vi "Process.vi"(8 "error in":errorcluster, 11 "Logger.Error":refnum<class "Logger.Error.lvclass">) -> (0 "error out":errorcluster, 3 "Logger.Error out":refnum<class "Logger.Error.lvclass">)   [LabVIEW 2019, in "Logger.Error.lvlib" / "Logger.Error.lvclass"]
doc: "---------------------------------------------------------------\nJKI State Machine Objects™\nhttp://jki.net/state-machine-objects/\nCopyright (C) 2005-2015, JKI <info@jki.net>\nALL RIGHTS RESERVED"
uses:
  Logger.Error.lvclass
  C:/Program Files/National Instruments/LabVIEW 2019/vi.lib/JKI/JKI SMO/SMO/SMO.lvclass
  Logger.Error.lvclass/Logger.Error.ctl
  <vilib>/JKI/JKI SMO/SMO/SMO.lvclass/SMO.ctl
  e2013399-adaa-4ae5-b634-22c116f18404.vi
  <vilib>/JKI/JKI SMO/SMO/Private/ReftoDVR--SMO.vi
  <vilib>/Utility/file.llb/Write Delimited Spreadsheet (string).vi
  <userlib>/LevyLab/Logger/Logger/Logger.lvclass
  <userlib>/LevyLab/Debug/Debug.lvlib
  <vilib>/JKI/JKI SMO/SMO/SMO.lvclass
panel:
  out "Status":string
  out "State History":string
  # "error Logger"
  # "For instructions on how to use the JKI State Machine Objects, examples and video tutorials, visit:\nhttp://jki.net/state-machine-objects/\n\nJKI State Machine Objects™\nhttp://jki.net/state-machine-objects/\nCopyright (C) 2005-2015, JKI <info@jki.net>\nALL RIGHTS RESERVED"
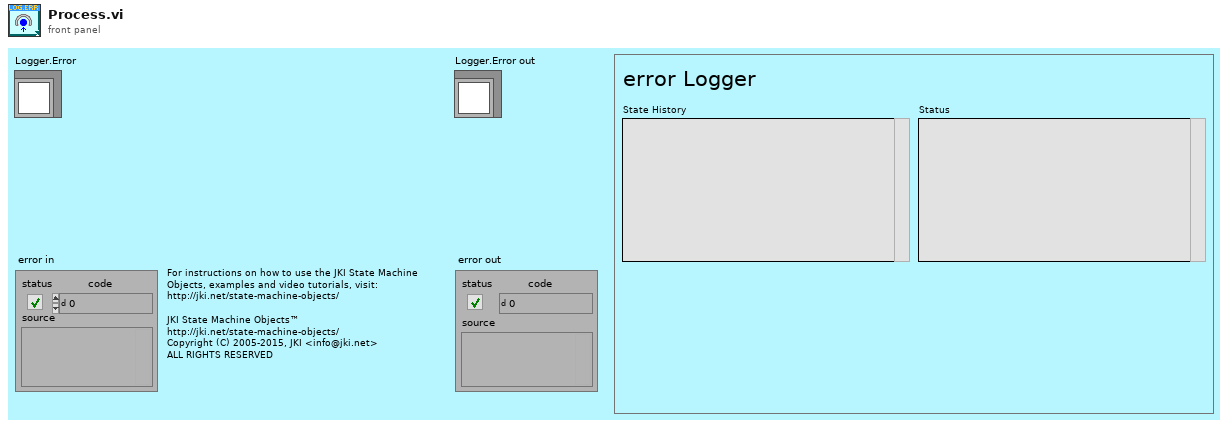
[diagram p1: front panel]
types:
  T1 = enum32{"invalid app kind", "Development System", "Run Time System", "Student Edition", "Embedded LabVIEW", "Evaluation", "Custom"}
  T2 = enum32{"Invalid", "Standard", "Closed", "Hidden", "Minimized", "Maximized"}
  T3 = cluster{"Core":cluster{"Current VI Reference":refnum<vi>, "Close Panel on Exit?":bool, "Last Error":cluster{"error":errorcluster, "previous state":string, "remaining states":string}, "Shutdown?":bool}, "SelfRef":refnum<class "Logger.Error.lvclass">, "path":path, "SMOs":refnum<class "SMO.lvclass">[], "error to log":errorcluster}
  T4 = cluster{"Current VI Reference":refnum<vi>, "Close Panel on Exit?":bool, "Last Error":cluster{"error":errorcluster, "previous state":string, "remaining states":string}, "Shutdown?":bool}
  T5 = typedef "Debug.lvlib/Attribute.Debug.lvclass/DebugBehavior.ctl" = enum16{"Normal", "Debug"}
  T6 = typedef "SMO.lvclass/Protected Events.ctl" = cluster{"StopProcesses":refnum<user-event>, "AbortProcesses":refnum<user-event>, "Config Changed":refnum<user-event>, "Dependency":refnum<user-event>}
  T7 = typedef "SMO.lvclass/Public Events.ctl" = cluster{"Error":refnum<user-event>, "State":refnum<user-event>, "Reserve State":refnum<user-event>}
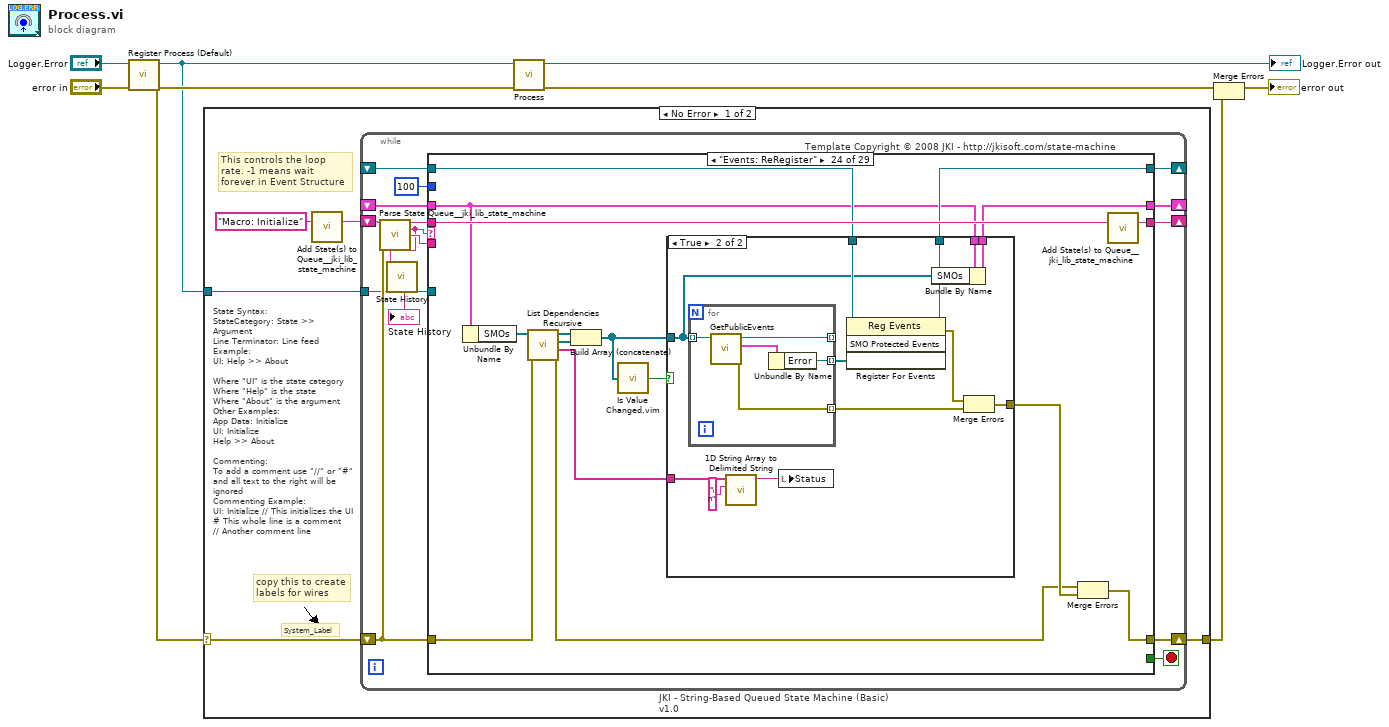
[diagram p0: block diagram]
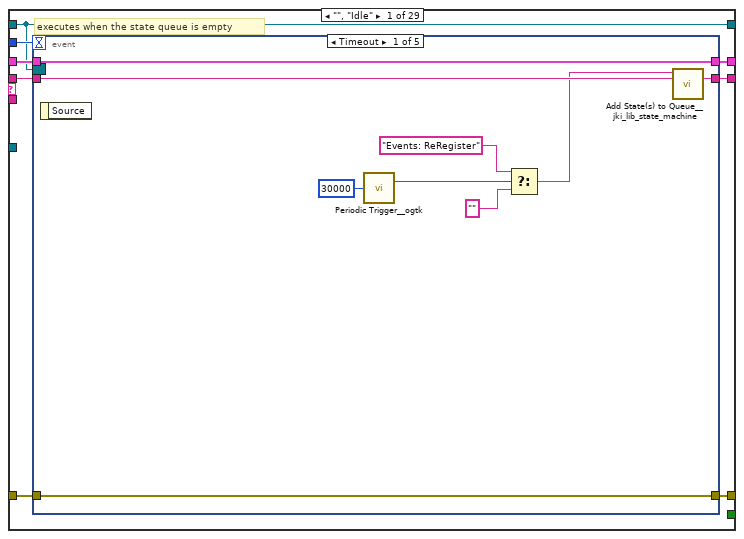
[diagram p2: hidden frame]
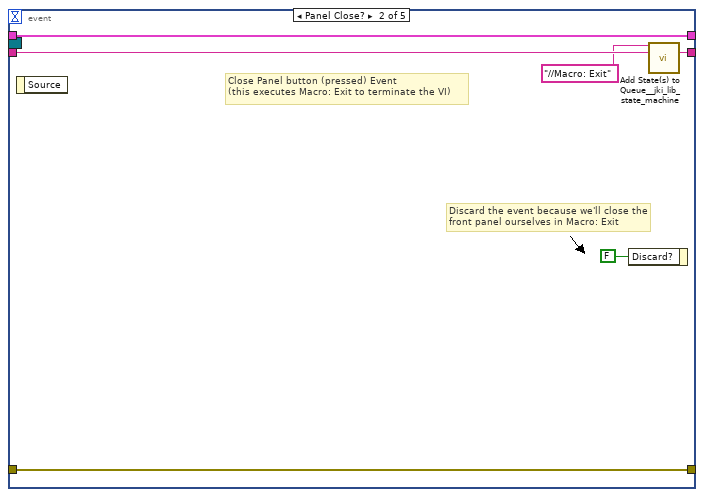
[diagram p3: hidden frame]
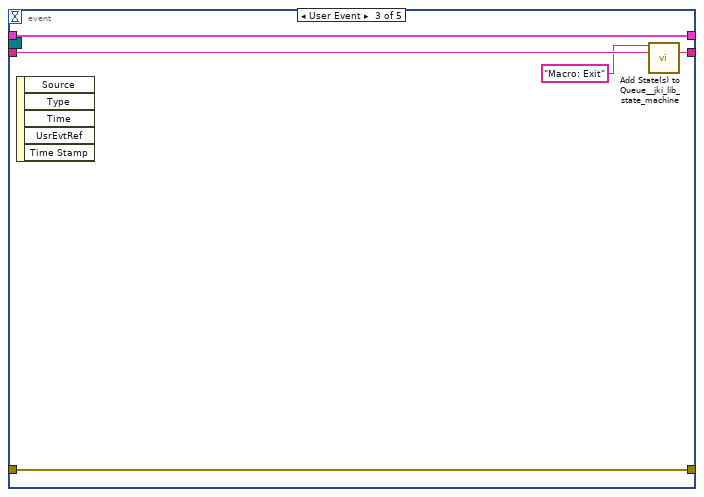
[diagram p4: hidden frame]
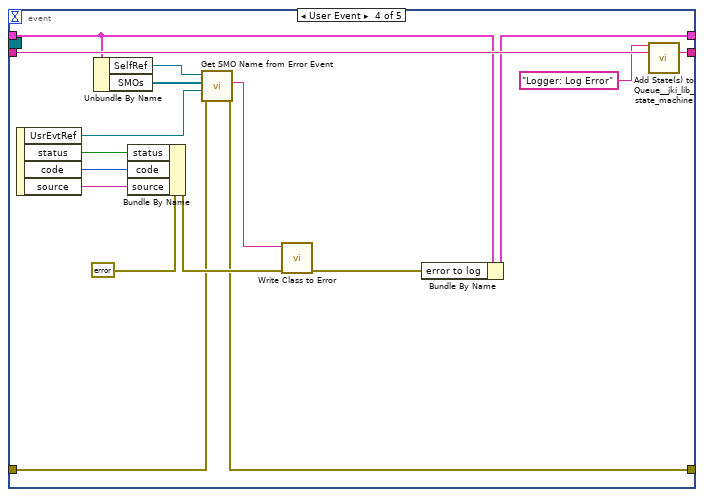
[diagram p5: hidden frame]
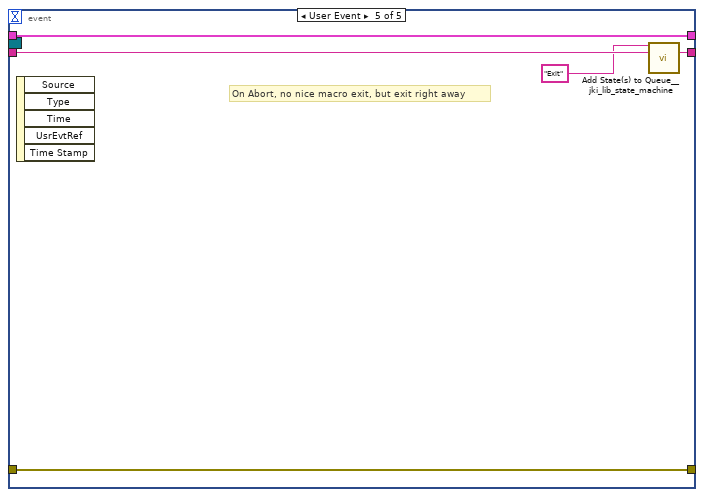
[diagram p6: hidden frame]
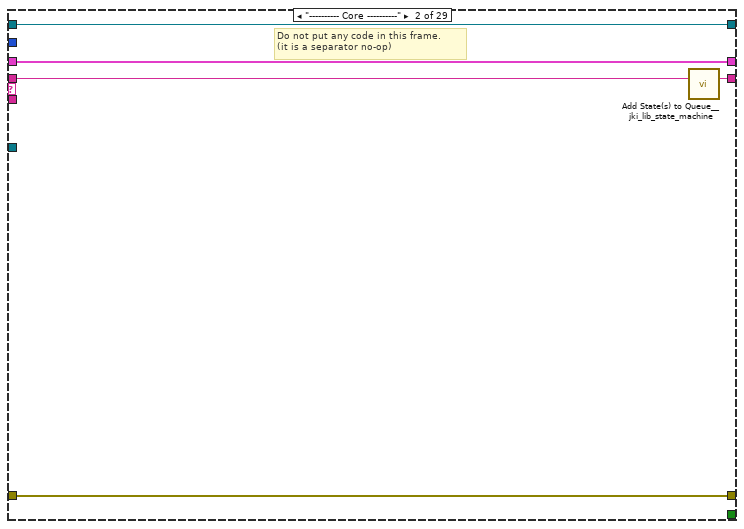
[diagram p7: hidden frame]
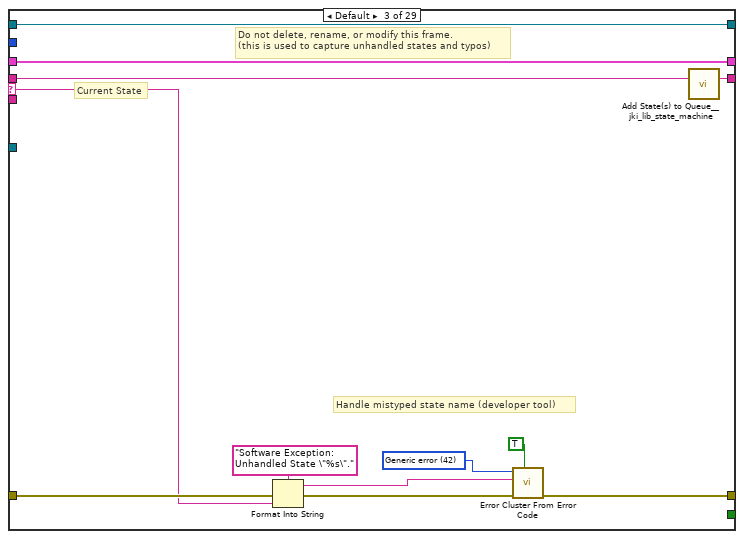
[diagram p8: hidden frame]
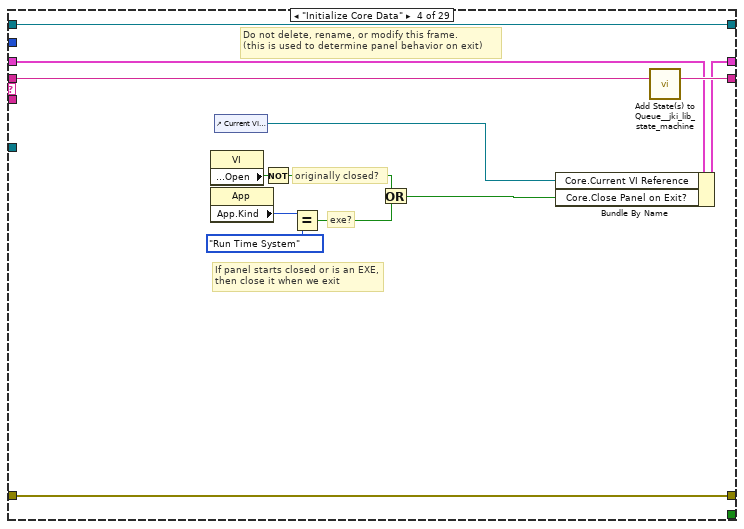
[diagram p9: hidden frame]
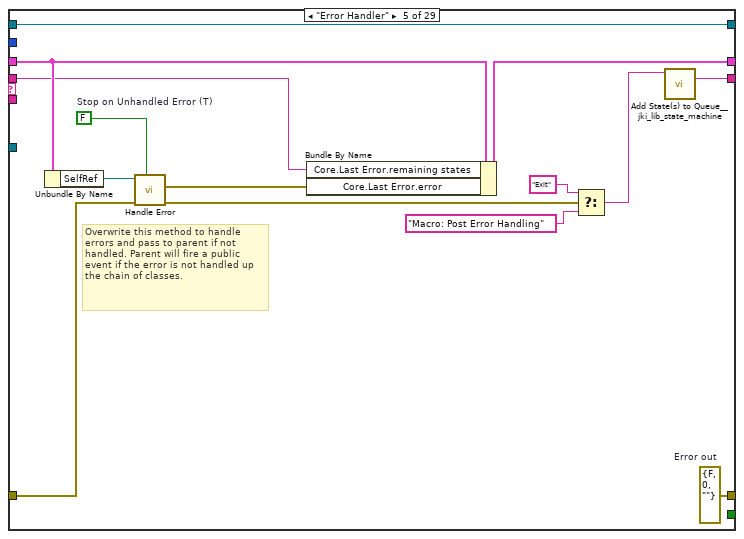
[diagram p10: hidden frame]
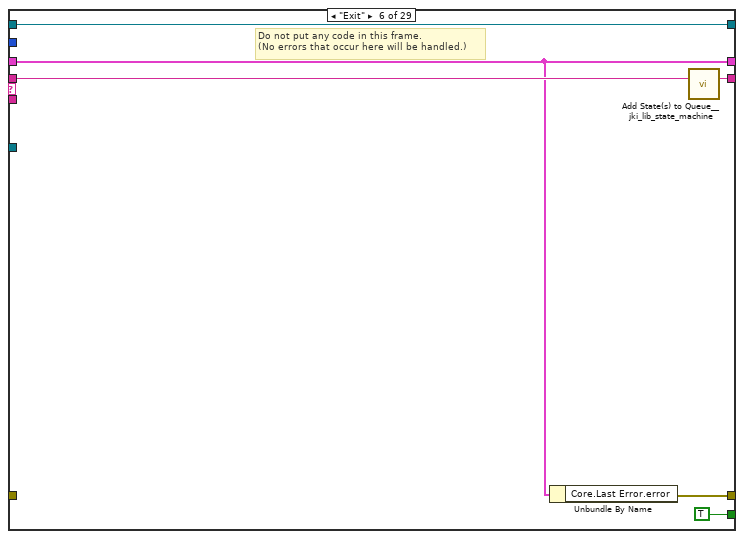
[diagram p11: hidden frame]
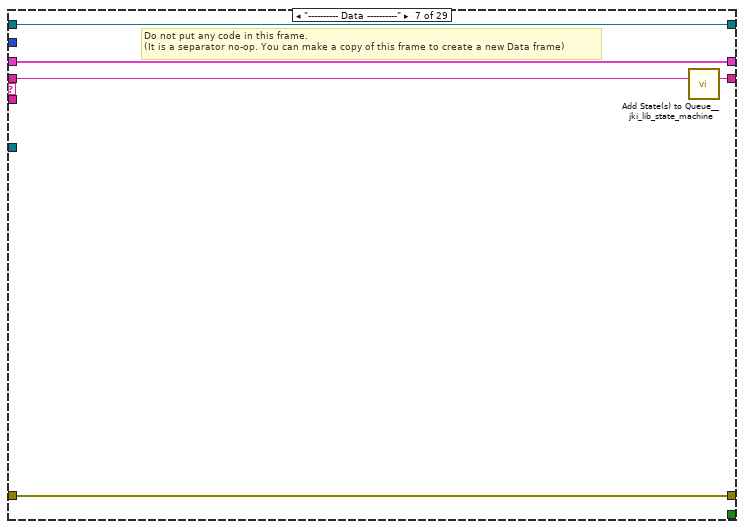
[diagram p12: hidden frame]
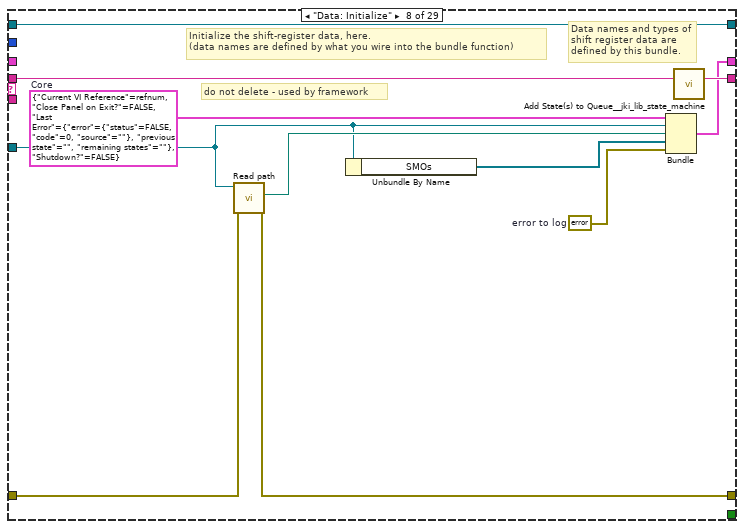
[diagram p13: hidden frame]
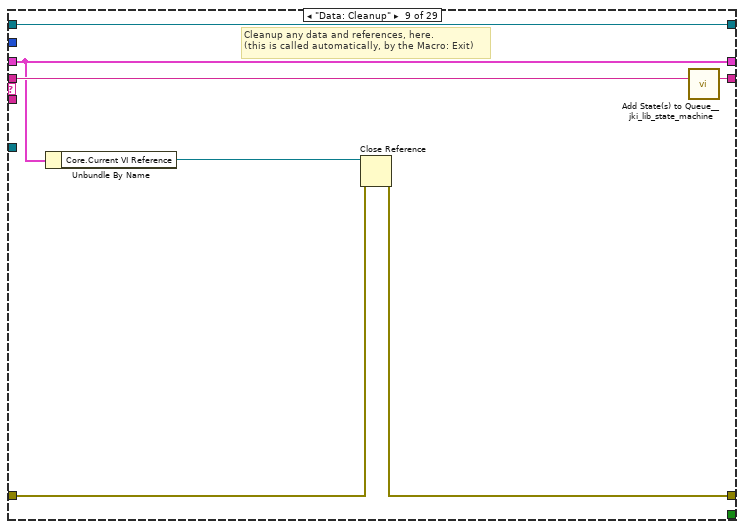
[diagram p14: hidden frame]
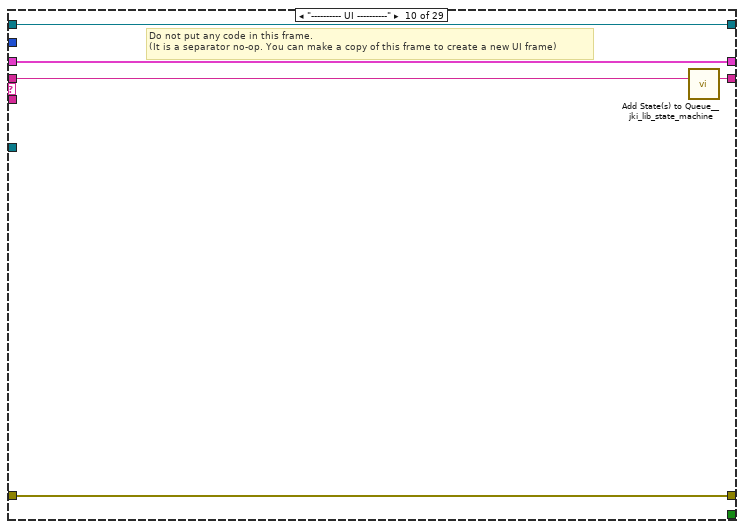
[diagram p15: hidden frame]
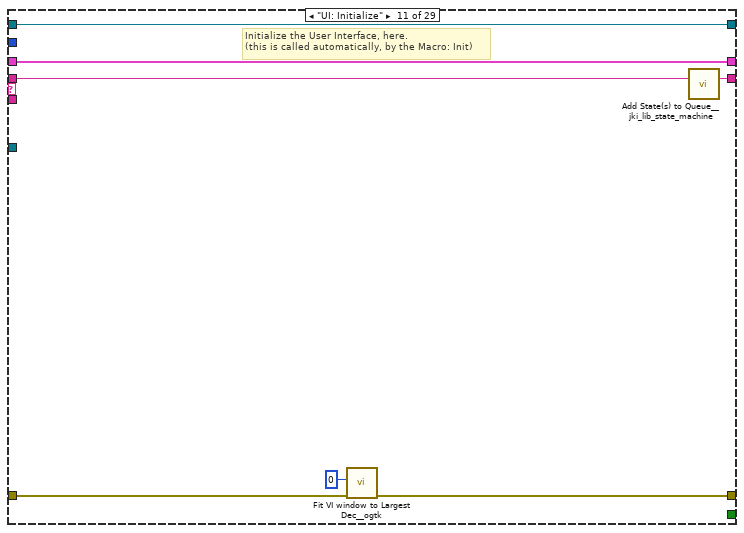
[diagram p16: hidden frame]
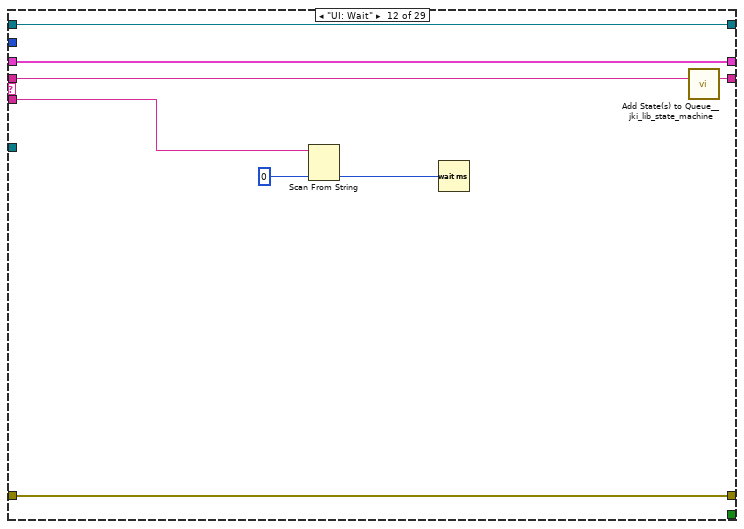
[diagram p17: hidden frame]
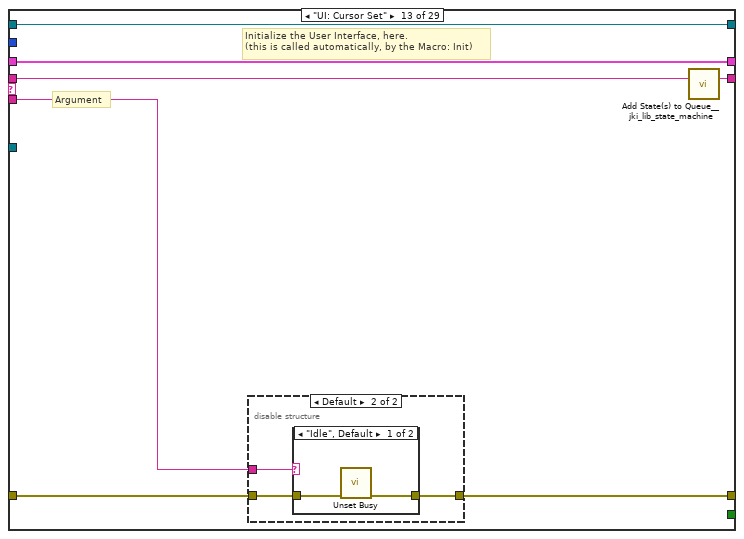
[diagram p18: hidden frame]
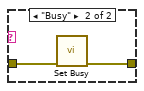
[diagram p20: hidden frame]
diagram:
  n1 = call <vilib>:"Register Process (Default).vi"("error in (no error)"="error in", "SMO"="Logger.Error") -> ("error out"=w5:errorcluster, "SelfRef"=w4:refnum<class "Logger.Error.lvclass">)  [unwired: 8 in]
  n2 = case shown="No Error" w5 {
    selector: w5 -> [w10 w420]
    tunnel: w4 -> [w11 _]
    tunnel: [w9 w420] -> w1
    frame No Error {
      # "State Syntax:\nStateCategory: State >> Argument\nLine Terminator: Line feed\nExample:\nUI: Help >> About\n\nWhere \"UI\" is the state category\nWhere \"Help\" is the state\nWhere \"About\" is the argument\nOther Examples:\nApp Data: Initialize\nUI: Initialize\nHelp >> About\n\nCommenting:\nTo add a comment use \"//\" or \"#\" and all text to the right will be ignored\nCommenting Example:\nUI: Initialize // This initializes the UI\n# This whole line is a comment\n// Another comment line"
      # "copy this to create labels for wires"
      # "This controls the loop rate. -1 means wait forever in Event Structure"
      # "System_Label"
      n3 = call <vilib>:"Add State(s) to Queue__jki_lib_state_machine.vi"("State(s) in (\"\")"="Macro: Initialize") -> ("States Out"=w13:string)  [unwired: 14 in]
      n4 = while "JKI - String-Based Queued State Machine (Basic) v1.0" {
        shift-right: [w22] -> _
        shift-left: _ -> [w14]
        shift-right: [w25] -> w9
        shift-left: w10 -> [w20]
        shift-right: [w24] -> _
        shift-left: w13 -> [w26]
        tunnel: w11 -> [w19]
        shift-right: [w18] -> _
        shift-left: _ -> [w17]
        stop <- w23 stop-if-true
        # "Template Copyright © 2008 JKI - http://jkisoft.com/state-machine"
        n5 = call <vilib>:"Parse State Queue__jki_lib_state_machine.vi"("State Queue"=w26, "Error In (no error)"=w20) -> ("Remaining States"=w28:string, "Current State"=w15:string, "Arguments"=w27:string)  [unwired: 11 in]
        n6 = call <userlib>:"State History.vi"("Current State"=w15) -> ("History"=→"State History":string)  [unwired: 10 in]
        n7 = case shown="\"Events: ReRegister\"" w15 {
          selector: w15 -> [_ _ w85 _ _ _ _ _ _ _ _ _ _ _ _ _ _ _ _ _ _ _ _ _ _ _ _ _ _]
          tunnel: w28 -> [w36 w83 w89 w108 w111 w128 w133 w144 w151 w156 w163 w171 w178 w194 w226 w238 w253 w270 w291 w296 w307 w312 w332 w356 w381 w386 w395 w402 w419]
          tunnel: w27 -> [_ _ _ _ _ _ _ _ _ _ _ w164 w172 w188 _ _ _ _ _ _ _ _ _ _ _ _ _ _ _]
          tunnel: [w33 w81 w91 w105 w118 w123 w131 w136 w147 w154 w158 w169 w173 w191 w224 w229 w240 w268 w289 w294 w299 w310 w328 w342 w377 w382 w391 w397 w404] -> w25
          tunnel: w20 -> [w32 w81 w90 w105 w119 _ w131 w137 w148 w154 w157 w169 w174 w192 w224 w229 w239 w268 w289 w294 w300 w310 w320 w343 w377 w382 w392 w398 w409]
          tunnel: [w35 w82 w88 w107 w122 w127 w132 w143 w150 w155 w162 w170 w177 w193 w225 w237 w252 w269 w290 w295 w306 w311 w331 w355 w380 w385 w394 w401 w418] -> w24
          tunnel: [_ _ _ _ _ TRUE _ _ _ _ _ _ _ _ _ _ _ _ _ _ _ _ _ _ _ _ _ _ _] -> w23
          tunnel: [w31 w80 w87 w106 w116 w124 w130 w142 w146 w153 w161 w168 w176 w190 w223 w231 w243 w260 w276 w293 w297 w309 w323 w347 w379 w384 w388 w396 w416] -> w22
          tunnel: 100 ("Timeout") -> [w30 _ _ _ _ _ _ _ _ _ _ _ _ _ _ _ _ _ _ _ _ _ _ _ _ _ _ _ _]
          tunnel: w19 -> [_ _ _ _ _ _ _ w135 _ _ _ _ _ _ _ _ _ _ _ _ _ _ _ _ _ _ _ _ _]
          tunnel: [w29 w79 w84 w96 w121 w125 w129 w141 w145 w152 w160 w167 w175 w187 w222 w236 w251 w267 w284 w292 w305 w308 w330 w348 w378 w383 w393 w400 w417] -> w18
          tunnel: w17 -> [w29 w79 w84 w96 w121 w125 w129 w141 w145 w152 w160 w167 w175 w187 w222 w236 w251 w267 w284 w292 w305 w308 _ w349 w378 w383 w393 w400 w417]
          tunnel: w14 -> [w34 w80 w87 w99 w117 w124 w130 _ w146 w153 w161 w168 w176 w190 w223 w231 w242 w259 w275 w293 w297 w309 w324 w346 w379 w384 w387 w396 w416]
          frame "", "Idle" {
            # "executes when the state queue is empty"
            n8 = event shown="[0] Timeout" {
              selector: w29 -> [_ _ _ _ _]
              dyn-events: _ -> [_ _ _ _ _]
              timeout: w30 -> [_ _ _ _ _]
              tunnel: w36 -> [w45 w51 w56 w73 w78]
              tunnel: [w44 w50 w55 w72 w77] -> w35
              tunnel: w34 -> [w42 w48 w53 w60 w75]
              tunnel: [w43 w49 w54 w62 w76] -> w33
              tunnel: w32 -> [w43 w49 w54 w63 w76]
              tunnel: [w42 w48 w53 w61 w75] -> w31
              event Timeout {
                n9 = event-data() -> ()  [unwired: 1 in, 1 out]
                n10 = call <userlib>:"Periodic Trigger__ogtk.vi"("time (ms)"=u32 30000) -> ("Triggered"=w39:bool)  [unwired: 12 in, 2 out]
                n11 = Select(t="Events: ReRegister", s=w39, f="") -> (s? t:f=w40:string)
                n12 = call <vilib>:"Add State(s) to Queue__jki_lib_state_machine.vi"("State(s) in Front (\"\")"=w40, "State(s) in (\"\")"=w45) -> ("States Out"=w44:string)  [unwired: 13 in]
              }
              event Panel Close? {
                # "Discard the event because we'll close the front panel ourselves in Macro: Exit"
                # "Close Panel button (pressed) Event\n(this executes Macro: Exit to terminate the VI)"
                n13 = event-data() -> ()  [unwired: 1 in, 1 out]
                n14 = event-data("Discard?"=FALSE) -> ()  [unwired: 1 in, 1 out]
                n15 = call <vilib>:"Add State(s) to Queue__jki_lib_state_machine.vi"("State(s) in Front (\"\")"="//Macro: Exit", "State(s) in (\"\")"=w51) -> ("States Out"=w50:string)  [unwired: 13 in]
              }
              event User Event {
                n16 = event-data() -> ()  [unwired: 1 in, 5 out]
                n17 = call <vilib>:"Add State(s) to Queue__jki_lib_state_machine.vi"("State(s) in Front (\"\")"="Macro: Exit", "State(s) in (\"\")"=w56) -> ("States Out"=w55:string)  [unwired: 13 in]
              }
              event User Event {
                n18 = event-data() -> ("UsrEvtRef"=w67:refnum<user-event>, "status"=w71:bool, "code"=w70:i32, "source"=w69:string)  [unwired: 1 in]
                n19 = Unbundle By Name(w60) -> ("SelfRef"=w57:refnum<class "Logger.Error.lvclass">, "SMOs"=w68:refnum<class "SMO.lvclass">[])
                n20 = Bundle By Name(cluster=errorcluster {"status"=FALSE, "code"=0, "source"=""} ("error in (no error)"), "status"=w71, "code"=w70, "source"=w69) -> (w65:errorcluster)
                n21 = call "Get SMO Name from Error Event.vi"("error in (no error)"=w63, "Error"=w67, "SMOs"=w68, "Logger.Error"=w57) -> ("error out"=w62:errorcluster, "class:SMO name"=w66:string)  [unwired: 5 in, 1 out]
                n22 = call "Write Class to Error.vi"("Error in"=w65, "Calling Class"=w66) -> ("Error out"=w59:errorcluster)  [unwired: 9 in]
                n23 = Bundle By Name(cluster=w60, "error to log"=w59) -> (w61:T3)
                n24 = call <vilib>:"Add State(s) to Queue__jki_lib_state_machine.vi"("State(s) in Front (\"\")"="Logger: Log Error" ("State(s) in Front (\"\")"), "State(s) in (\"\")"=w73) -> ("States Out"=w72:string)  [unwired: 13 in]
              }
              event User Event {
                # "On Abort, no nice macro exit, but exit right away"
                n25 = event-data() -> ()  [unwired: 1 in, 5 out]
                n26 = call <vilib>:"Add State(s) to Queue__jki_lib_state_machine.vi"("State(s) in Front (\"\")"="Exit", "State(s) in (\"\")"=w78) -> ("States Out"=w77:string)  [unwired: 13 in]
              }
            }
          }
          frame "---------- Core ----------" {
            # "Do not put any code in this frame.\n(it is a separator no-op)"
            n27 = call <vilib>:"Add State(s) to Queue__jki_lib_state_machine.vi"("State(s) in (\"\")"=w83) -> ("States Out"=w82:string)  [unwired: 14 in]
          }
          frame Default {
            w94 = 42 items=["No error", "Argument error", "Memory is full", "Out of zone", "End of file", "File already open", "Generic file I/O error", "File not found", "File permission error", "Disk is full", "Duplicate path", "Too many files open", "System feature not enabled", "Resource file not found", "Cannot add resource", "Resource not found", "Image not found", "Image memory error", "Pen does not exist", "Config type invalid", "Config token not found", "Config parse error", "Config memory error", "Bad external code format", "Bad external code offset", "External code not present", "Null window", "Destroy window error", "Null menu", "Print aborted", "Bad print record", "Print driver error", "Windows error during printing", "Memory error during printing", "Print dialog error", "Generic print error", "Invalid device refnum", "Device not found", "Device parameter error", "Device unit error", "Cannot open device", "Device call aborted", "Generic error", "Cancelled by user", "Object ID too low", "Object ID too high", "Object not in heap", "Unknown heap", "Unknown object (invalid DefProc)", "Unknown object (DefProc not in table)", "Message out of range", "Invalid (null) method", "Unknown message", "Manager call not supported", "Bad address", "Network operation in progress", "Network operation timed out", "Connection is busy", "Network attribute not supported", "Network error", "Address in use", "System out of memory", "Connection aborted", "Connection refused", "Not connected", "Already connected", "Connection closed", "Initialization error (interapplication manager)", "Bad occurrence", "Wait on unbound occurrence handler", "Occurrence queue overflow", "Datalog type conflict", "Unused", "Unrecognized type (interapplication manager)", "Memory corrupt", "Failed to make temporary DLL", "Old CIN version", "Drag socket not found", "Failed to load drop-object", "Failed to register OLE object", "Failed to release OLE object", "Format specifier type mismatch", "Unknown format specifier", "Too few format specifiers", "Too many format specifiers", "Scan failed", "Newer CIN version", "Error converting to variant", "Runtime menu error", "Password tampered", "Variant attribute not found", "Incompatible variant data type", "Event data is not available", "Event Store is not present", "Occurrence is not found", "Event Queue is not created", "Event info is not available", "Refnum passed is NULL", "Error retrieving Class GUID", "Error retrieving CoClass GUID", "Error retrieving TypeLib GUID.", "Bad built application magic bytes.", "Specific driver is different from the specific driver associated with the Logical Name.", "There is no session opened to the class driver.", "Max Error", "MAX - Error with config objects", "MAX - Error loading configuration", "MAX - Group not supported"]
            # "Current State"
            # "Do not delete, rename, or modify this frame.\n(this is used to capture unhandled states and typos)"
            # "Handle mistyped state name (developer tool)"
            n28 = Format Into String(format string="Software Exception: Unhandled State \"%s\"." ("message"), error in=w90, w85) -> (resulting string=w93:string, error out=w92:errorcluster)  [unwired: 1 in]
            n29 = call <vilib>:"Error Cluster From Error Code.vi"("show call chain? (False)"=TRUE, "error in (no error)"=w92, "error message (\"\")"=w93, "error code (0)"=w94) -> ("error out"=w91:errorcluster)  [unwired: 5 in]
            n30 = call <vilib>:"Add State(s) to Queue__jki_lib_state_machine.vi"("State(s) in (\"\")"=w89) -> ("States Out"=w88:string)  [unwired: 14 in]
          }
          frame "Initialize Core Data" {
            # "Do not delete, rename, or modify this frame.\n(this is used to determine panel behavior on exit)"
            # "originally closed?"
            # "exe?"
            # "If panel starts closed or is an EXE, then close it when we exit"
            n31 = property class="VI"() -> ("Front Panel.Open"=w104:bool)  [unwired: 2 in, 2 out]
            n32 = property class="App"() -> ("App.Kind"=w103:T1)  [unwired: 2 in, 2 out]
            n33 = control-ref of="Current VI Reference"() -> (w97:refnum<vi>)
            n34 = Not(x=w104) -> (.not. x?=w101:bool)
            n35 = Equal?(x=w103, y=T1."Run Time System" ("Application:Kind")) -> (x = y?=w100:bool)
            n36 = Or(x=w101, y=w100) -> (x .or. y?=w98:bool)
            n37 = Bundle By Name(cluster=w99, "Core.Current VI Reference"=w97, "Core.Close Panel on Exit?"=w98) -> (w106:T3)
            n38 = call <vilib>:"Add State(s) to Queue__jki_lib_state_machine.vi"("State(s) in (\"\")"=w108) -> ("States Out"=w107:string)  [unwired: 14 in]
          }
          frame "Error Handler" {
            w112 = FALSE  # Stop on Unhandled Error (T)
            w118 = errorcluster {"status"=FALSE, "code"=0, "source"=""}  # Error out
            # "Overwrite this method to handle errors and pass to parent if not handled. Parent will fire a public event if the error is not handled up the chain of classes."
            n39 = Unbundle By Name(w117) -> ("SelfRef"=w120:refnum<class "Logger.Error.lvclass">)
            n40 = call-dynamic "Handle Error.vi"("Stop on Unhandled Error (T)"=w112, "error in"=w119, "SMO"=w120) -> ("handling error"=w113:errorcluster, "Unhandled error"=w109:errorcluster)  [unwired: 6 in, 1 out]
            n41 = Bundle By Name(cluster=w117, "Core.Last Error.remaining states"=w111, "Core.Last Error.error"=w109) -> (w116:T3)
            n42 = Select(t="Exit", s=w113, f="Macro: Post Error Handling") -> (s? t:f=w115:string)
            n43 = call <vilib>:"Add State(s) to Queue__jki_lib_state_machine.vi"("State(s) in Front (\"\")"=w115) -> ("States Out"=w122:string)  [unwired: 14 in]
          }
          frame "Exit" {
            # "Do not put any code in this frame.\n(No errors that occur here will be handled.)"
            n44 = Unbundle By Name(w124) -> ("Core.Last Error.error"=w123:errorcluster)
            n45 = call <vilib>:"Add State(s) to Queue__jki_lib_state_machine.vi"("State(s) in (\"\")"=w128) -> ("States Out"=w127:string)  [unwired: 14 in]
          }
          frame "---------- Data ----------" {
            # "Do not put any code in this frame.\n(It is a separator no-op. You can make a copy of this frame to create a new Data frame)"
            n46 = call <vilib>:"Add State(s) to Queue__jki_lib_state_machine.vi"("State(s) in (\"\")"=w133) -> ("States Out"=w132:string)  [unwired: 14 in]
          }
          frame "Data: Initialize" {
            w138 = errorcluster {"status"=FALSE, "code"=0, "source"=""}  # error to log
            w140 = T4 {"Current VI Reference"=refnum, "Close Panel on Exit?"=FALSE, "Last Error"={"error"={"status"=FALSE, "code"=0, "source"=""}, "previous state"="", "remaining states"=""}, "Shutdown?"=FALSE}  # Core
            # "do not delete - used by framework"
            # "Data names and types of shift register data are defined by this bundle."
            # "Initialize the shift-register data, here.\n(data names are defined by what you wire into the bundle function)"
            n47 = call-dynamic "Read path.vi"("error in (no error)"=w137, "Logger in"=w135) -> ("error out"=w136:errorcluster, "path"=w139:path)  [unwired: 7 in, 1 out]
            n48 = Unbundle By Name(w135) -> ("SMOs"=w134:refnum<class "SMO.lvclass">[])
            n49 = Bundle("Core"=w140, "SelfRef"=w135, "path"=w139, "SMOs"=w134, "error to log"=w138) -> (w142:T3)  [unwired: 1 in]
            n50 = call <vilib>:"Add State(s) to Queue__jki_lib_state_machine.vi"("State(s) in (\"\")"=w144) -> ("States Out"=w143:string)  [unwired: 14 in]
          }
          frame "Data: Cleanup" {
            # "Cleanup any data and references, here.\n(this is called automatically, by the Macro: Exit)"
            n51 = Unbundle By Name(w146) -> ("Core.Current VI Reference"=w149:refnum<vi>)
            n52 = Close Reference(reference=w149, error in (no error)=w148) -> (error out=w147:errorcluster)
            n53 = call <vilib>:"Add State(s) to Queue__jki_lib_state_machine.vi"("State(s) in (\"\")"=w151) -> ("States Out"=w150:string)  [unwired: 14 in]
          }
          frame "---------- UI ----------" {
            # "Do not put any code in this frame.\n(It is a separator no-op. You can make a copy of this frame to create a new UI frame)"
            n54 = call <vilib>:"Add State(s) to Queue__jki_lib_state_machine.vi"("State(s) in (\"\")"=w156) -> ("States Out"=w155:string)  [unwired: 14 in]
          }
          frame "UI: Initialize" {
            # "Initialize the User Interface, here.\n(this is called automatically, by the Macro: Init)"
            n55 = call <userlib>:"Fit VI window to Largest Dec__ogtk.vi"("error in (no error)"=w157, "border spacing (2 px)"=0) -> ("error out"=w158:errorcluster)  [unwired: 4 in, 1 out]
            n56 = call <vilib>:"Add State(s) to Queue__jki_lib_state_machine.vi"("State(s) in (\"\")"=w163) -> ("States Out"=w162:string)  [unwired: 14 in]
          }
          frame "UI: Wait" {
            n57 = Scan From String(input string=w164, default 1=u32 0) -> (output 1=w165:u32)  [unwired: 3 in, 3 out]
            n58 = Wait (ms)(milliseconds to wait=w165) -> ()  [unwired: 1 out]
            n59 = call <vilib>:"Add State(s) to Queue__jki_lib_state_machine.vi"("State(s) in (\"\")"=w171) -> ("States Out"=w170:string)  [unwired: 14 in]
          }
          frame "UI: Cursor Set" {
            # "Argument"
            # "Initialize the User Interface, here.\n(this is called automatically, by the Macro: Init)"
            n60 = disable-structure shown="Default" {
              disable-tunnel: w174 -> [w179 w182]
              disable-tunnel: [w179 w181] -> w173
              disable-tunnel: w172 -> [_ w180]
              frame condition #0 {
              }
              frame condition #1 (active) {
                n61 = case shown="\"Idle\", Default" w180 {
                  tunnel: w182 -> [w184 w186]
                  tunnel: [w183 w185] -> w181
                  frame "Idle", Default {
                    n62 = call <vilib>:"Unset Busy.vi"("error in (no error)"=w184) -> ("error out"=w183:errorcluster)  [unwired: 10 in]
                  }
                  frame "Busy" {
                    n63 = call <vilib>:"Set Busy.vi"("error in (no error)"=w186) -> ("error out"=w185:errorcluster)  [unwired: 9 in, 1 out]
                  }
                }
              }
            }
            n64 = call <vilib>:"Add State(s) to Queue__jki_lib_state_machine.vi"("State(s) in (\"\")"=w178) -> ("States Out"=w177:string)  [unwired: 14 in]
          }
          frame "UI: Front Panel State" {
            # "Argument"
            # "Set Front Panel Open or Closed\n(Usage: \"UI: Front Panel State >> Open|Close\")"
            n65 = Unbundle By Name(w190) -> ("Core.Current VI Reference"=w189:refnum<vi>)
            n66 = disable-structure shown="Default" {
              disable-tunnel: w192 -> [w198 w221]
              disable-tunnel: [w197 w221] -> w191
              disable-tunnel: w189 -> [w196 _]
              disable-tunnel: w188 -> [w195 _]
              frame condition #0 (active) {
                n67 = case shown="\"Close\"" w195 {
                  tunnel: w198 -> [w202 w215]
                  tunnel: [w204 w216] -> w197
                  tunnel: w196 -> [w203 w213]
                  frame "Open", Default {
                    n68 = property class="VI"(reference=w203, error in=w202) -> (reference out=w200:refnum<vi>, error out=w201:errorcluster, "FP.State"=w199:T2)
                    n69 = case shown="\"Closed\"" w199 {
                      tunnel: [w207 w210] -> w204
                      tunnel: w201 -> [w206 w210]
                      tunnel: w200 -> [w205 _]
                      frame "Closed" {
                        n70 = invoke class="VI" method="FP.Open"(reference=w205, error in=w206, "Activate"=TRUE, "State"=T2."Standard") -> (error out=w207:errorcluster)  [unwired: 1 in, 4 out]
                      }
                      frame Default {
                      }
                    }
                  }
                  frame "Close" {
                    n71 = property class="VI"(reference=w213, error in=w215) -> (reference out=w212:refnum<vi>, error out=w214:errorcluster, "FP.State"=w211:T2)
                    n72 = case shown="Default" w211 {
                      tunnel: [w217 w220] -> w216
                      tunnel: w214 -> [w217 w219]
                      tunnel: w212 -> [_ w218]
                      frame "Invalid", "Closed" {
                      }
                      frame Default {
                        n73 = invoke class="VI" method="FP.Close"(reference=w218, error in=w219) -> (error out=w220:errorcluster)  [unwired: 1 in, 2 out]
                      }
                    }
                  }
                }
              }
              frame condition #1 {
              }
            }
            n74 = call <vilib>:"Add State(s) to Queue__jki_lib_state_machine.vi"("State(s) in (\"\")"=w194) -> ("States Out"=w193:string)  [unwired: 14 in]
          }
          frame "---------- Macro ----------" {
            # "Do not put any code in this frame.\n(It is a separator no-op. You can make a copy of this frame to create a new Macro frame)"
            n75 = call <vilib>:"Add State(s) to Queue__jki_lib_state_machine.vi"("State(s) in (\"\")"=w226) -> ("States Out"=w225:string)  [unwired: 14 in]
          }
          frame "Macro: Initialize" {
            w227 = "UI: Wait >> 1000\nEvents: ReRegister"  # UI: Wait >> 1000 Events: ReRegister
            # "Initialization Macro\n(This is called once, when the VI starts)"
            n76 = call <vilib>:"Add State(s) to Queue__jki_lib_state_machine.vi"("State(s) in Front (\"\")"="UI: Initialize", "State(s) in (\"\")"="UI: Front Panel State >> Close\nMacro: Debug\nLogger: Start Error Logger", "State(s) at Back (\"\")"=w227) -> ("States Out"=w230:string)  [unwired: 12 in]
            n77 = call <vilib>:"Add State(s) to Queue__jki_lib_state_machine.vi"("State(s) in Front (\"\")"="Data: Initialize\nInitialize Core Data\nEvents: Register", "State(s) in (\"\")"="Process: Sync", "State(s) at Back (\"\")"=w230) -> ("States Out"=w234:string)  [unwired: 12 in]
            n78 = call <vilib>:"Add State(s) to Queue__jki_lib_state_machine.vi"("State(s) in Front (\"\")"=w234, "State(s) in (\"\")"=w238) -> ("States Out"=w237:string)  [unwired: 13 in]
          }
          frame "Macro: Debug" {
            # "exe?"
            # "If pane is an EXE, then close it when we exit"
            # "Macro: Debug\n(get debug behavior, determine UI and determine shutdown behavior)"
            n79 = Unbundle By Name(w242) -> ("Core.Close Panel on Exit?"=w245:bool, "SelfRef"=w250:refnum<class "Logger.Error.lvclass">)
            n80 = property class="App"() -> ("App.Kind"=w248:T1)  [unwired: 2 in, 2 out]
            n81 = Equal?(x=w248, y=T1."Run Time System" ("Application:Kind")) -> (x = y?=w244:bool)
            n82 = call <userlib>:"Get Debug Mode.vi"("error in (no error)"=w239, "SMO"=w250) -> ("error out"=w240:errorcluster, "Behavior"=w249:T5)  [unwired: 7 in, 1 out]
            n83 = case shown="\"Debug\"" w249 {
              tunnel: [w254 w256] -> w246
              tunnel: w245 -> [w254 _]
              tunnel: w244 -> [_ w258]
              tunnel: [_ "UI: Front Panel State >> Open\nUI: Wait >> 1000"] -> w241
              frame "Normal", Default {
                # "respect core.close"
              }
              frame "Debug" {
                # "keep panel open\nunless exe"
                n84 = Or(x=w258, y=FALSE) -> (x .or. y?=w256:bool)
              }
            }
            n85 = Bundle By Name(cluster=w242, "Core.Close Panel on Exit?"=w246) -> (w243:T3)
            n86 = call <vilib>:"Add State(s) to Queue__jki_lib_state_machine.vi"("State(s) in Front (\"\")"=w241, "State(s) in (\"\")"=w253) -> ("States Out"=w252:string)  [unwired: 13 in]
          }
          frame "Macro: Post Error Handling" {
            # "Clear Last Error?"
            n87 = Unbundle By Name(w259) -> ("Core.Last Error.remaining states"=w262:string, "Core.Shutdown?"=w263:bool)
            n88 = Unbundle By Name(w259) -> ("Core.Last Error.error"=w266:errorcluster)
            n89 = case shown="False" FALSE {
              tunnel: w266 -> [w274 _]
              tunnel: [w274 _] -> w265
              frame False {
              }
              frame True {
              }
            }
            n90 = case shown="True" w263 {
              tunnel: w262 -> [w271 w273]
              tunnel: [w271 w272] -> w261
              frame False {
                # "These are the remaining states (at the moment the error occured). States can be altered according to business logic."
                # "NOT SHUTTING DOWN"
              }
              frame True {
                # "Developer can decide to alter the states but should be aware that during the shutdown process, there are certain states that must be run for the SMO to properly shut itself (and this process) down. As such, one can add states to perform additional clean-ups, but should append the remaining state to be executed."
                # "SHUTTING DOWN"
                n91 = call <vilib>:"Add State(s) to Queue__jki_lib_state_machine.vi"("State(s) in (\"\")"=w273) -> ("States Out"=w272:string)  [unwired: 14 in]
              }
            }
            n92 = Bundle By Name(cluster=w259, "Core.Last Error.error"=w265) -> (w260:T3)
            n93 = call <vilib>:"Add State(s) to Queue__jki_lib_state_machine.vi"("State(s) in Front (\"\")"=w261, "State(s) in (\"\")"=w270) -> ("States Out"=w269:string)  [unwired: 13 in]
          }
          frame "Macro: Exit" {
            # "Exit Macro\n(This is called once, when the VI exits)"
            n94 = Unbundle By Name(w275) -> ("Core.Close Panel on Exit?"=w288:bool)
            n95 = Bundle By Name(cluster=w275, "Core.Shutdown?"=TRUE) -> (w276:T3)
            n96 = Select(t="UI: Front Panel State >> Close", s=w288, f="") -> (s? t:f=w286:string)
            n97 = call <vilib>:"Add State(s) to Queue__jki_lib_state_machine.vi"("State(s) in Front (\"\")"="Logger: Stop Error Logger\nData: Cleanup\nEvents: Unregister", "State(s) in (\"\")"="Process: Sync", "State(s) at Back (\"\")"="Exit") -> ("States Out"=w281:string)  [unwired: 12 in]
            n98 = call <vilib>:"Add State(s) to Queue__jki_lib_state_machine.vi"("State(s) in Front (\"\")"="" ("State(s) in Front (\"\")"), "State(s) in (\"\")"=w286, "State(s) at Back (\"\")"=w281) -> ("States Out"=w285:string)  [unwired: 12 in]
            n99 = call <vilib>:"Add State(s) to Queue__jki_lib_state_machine.vi"("State(s) in Front (\"\")"=w285, "State(s) in (\"\")"=w291) -> ("States Out"=w290:string)  [unwired: 13 in]
          }
          frame "---------- Process ----------" {
            # "Template Separator\n(You can make a copy of, or modify, this frame)"
            n100 = call <vilib>:"Add State(s) to Queue__jki_lib_state_machine.vi"("State(s) in (\"\")"=w296) -> ("States Out"=w295:string)  [unwired: 14 in]
          }
          frame "Process: Sync" {
            n101 = Unbundle By Name(w297) -> ("SelfRef"=w301:refnum<class "Logger.Error.lvclass">)
            n102 = call <vilib>:"WaitOnProcessSync.vi"("error in (no error)"=w300, "SMO"=w301) -> ("error out"=w299:errorcluster, "Don't run?"=w304:bool)  [unwired: 7 in, 1 out]
            n103 = Select(t="Data: Cleanup\nEvents: Unregister\nExit", s=w304, f="") -> (s? t:f=w298:string)
            n104 = call <vilib>:"Add State(s) to Queue__jki_lib_state_machine.vi"("State(s) in Front (\"\")"=w298, "State(s) in (\"\")"=w307) -> ("States Out"=w306:string)  [unwired: 13 in]
          }
          frame "---------- Events ----------" {
            # "Template Separator\n(You can make a copy of, or modify, this frame)"
            n105 = call <vilib>:"Add State(s) to Queue__jki_lib_state_machine.vi"("State(s) in (\"\")"=w312) -> ("States Out"=w311:string)  [unwired: 14 in]
          }
          frame "Events: Register" {
            n106 = Unbundle By Name(w324) -> ("SelfRef"=w329:refnum<class "Logger.Error.lvclass">)
            n107 = call <vilib>:"GetProtectedEvents.vi"("SMO"=w329) -> ("error out"=w327:errorcluster, "SMO Protected Events"=w326:T6, "SMO out"=w325:refnum<class "Logger.Error.lvclass">)  [unwired: 8 in]
            n108 = Unbundle By Name(w325) -> ("SMOs"=w318:refnum<class "SMO.lvclass">[])
            n109 = Build Array (concatenate)(w318, w325) -> (w316:refnum<class "SMO.lvclass">[])
            n110 = for {
              tunnel: w316 -> [w335] mode=indexing
              tunnel: [w339] -> w322 mode=indexing
              tunnel: [w337] -> w321 mode=indexing
              tunnel: [w338] -> w317 mode=indexing
              tunnel: [w333] -> w313 mode=indexing
              n111 = call <vilib>:"GetName.vi"("SMO"=w335) -> ("error out"=w334:errorcluster, "Name"=w333:string, "SMO out"=w336:refnum<class "SMO.lvclass">)  [unwired: 7 in, 1 out]
              n112 = call <vilib>:"GetPublicEvents.vi"("error in (no error)"=w334, "SMO"=w336) -> ("error out"=w338:errorcluster, "Public Events"=w340:T7, "SMO out"=w337:refnum<class "SMO.lvclass">)  [unwired: 7 in]
              n113 = Unbundle By Name(w340) -> ("Error"=w339:refnum<user-event>)
            }
            n114 = register-events(w326, w322) -> (reference out=w330:refnum<event-registration>, error out=w319:errorcluster)  [unwired: 2 in]
            n115 = call <vilib>:"1D String Array to Delimited String.vi"("delimiter"="\n", "string array"=w313) -> ("delimited string"=w315:string)  [unwired: 9 in]
            n116 = local write "Status"(w315) -> ()
            n117 = Bundle By Name(cluster=w324, "SMOs"=w321) -> (w323:T3)
            n118 = Merge Errors(w319, w317, w327, w320) -> (w328:errorcluster)
            n119 = call <vilib>:"Add State(s) to Queue__jki_lib_state_machine.vi"("State(s) in (\"\")"=w332) -> ("States Out"=w331:string)  [unwired: 14 in]
          }
          frame "Events: ReRegister" {
            n120 = Unbundle By Name(w346) -> ("SMOs"=w350:refnum<class "SMO.lvclass">[])
            n121 = call "List Dependencies Recursive.vi"("error in (no error)"=w343, "SMOs in"=w350) -> ("error out"=w344:errorcluster, "Names"=w341:string[], "[Dependencies]"=w353:refnum<class "SMO.lvclass">[], "SMOs out"=w354:refnum<class "SMO.lvclass">[])  [unwired: 6 in]
            n122 = Build Array (concatenate)(w354, w353) -> (w352:refnum<class "SMO.lvclass">[])
            n123 = call "Is Value Changed.vim"("value"=w352) -> ("changed or first call?"=w351:bool)
            n124 = case shown="True" w351 {
              tunnel: [w358 w370] -> w348
              tunnel: w352 -> [_ w364]
              tunnel: w349 -> [w358 w367]
              tunnel: [_ w365] -> w345
              tunnel: w346 -> [w357 w363]
              tunnel: [w357 w362] -> w347
              tunnel: w341 -> [_ w361]
              frame False {
              }
              frame True {
                n125 = for {
                  tunnel: w364 -> [w374] mode=indexing
                  tunnel: [w373] -> w369 mode=indexing
                  tunnel: [w371] -> _ mode=indexing
                  tunnel: [w372] -> w368 mode=indexing
                  n126 = call <vilib>:"GetPublicEvents.vi"("SMO"=w374) -> ("error out"=w372:errorcluster, "Public Events"=w375:T7, "SMO out"=w371:refnum<class "SMO.lvclass">)  [unwired: 8 in]
                  n127 = Unbundle By Name(w375) -> ("Error"=w373:refnum<user-event>)
                }
                n128 = call <vilib>:"1D String Array to Delimited String.vi"("delimiter"="\n", "string array"=w361) -> ("delimited string"=w359:string)  [unwired: 9 in]
                n129 = local write "Status"(w359) -> ()
                n130 = register-events(reference=w367, w369) -> (reference out=w370:refnum<event-registration>, error out=w366:errorcluster)  [unwired: 2 in]
                n131 = Bundle By Name(cluster=w363, "SMOs"=w364) -> (w362:T3)
                n132 = Merge Errors(w366, w368) -> (w365:errorcluster)
              }
            }
            n133 = Merge Errors(w344, w345) -> (w342:errorcluster)
            n134 = call <vilib>:"Add State(s) to Queue__jki_lib_state_machine.vi"("State(s) in (\"\")"=w356) -> ("States Out"=w355:string)  [unwired: 14 in]
          }
          frame "Events: Unregister" {
            n135 = Unregister For Events(event registration refnum=w378, error in=w377) -> (error out=w376:errorcluster)
            n136 = call <vilib>:"Clear Errors.vi"("error in (no error)"=w376) -> ()  [unwired: 5 in, 2 out]
            n137 = call <vilib>:"Add State(s) to Queue__jki_lib_state_machine.vi"("State(s) in (\"\")"=w381) -> ("States Out"=w380:string)  [unwired: 14 in]
          }
          frame "---------- Logger ----------" {
            n138 = call <vilib>:"Add State(s) to Queue__jki_lib_state_machine.vi"("State(s) in (\"\")"=w386) -> ("States Out"=w385:string)  [unwired: 14 in]
          }
          frame "Logger: Start Error Logger" {
            # "will these work with other SMOs?"
            n139 = Unbundle By Name(w387) -> ("SelfRef"=w390:refnum<class "Logger.Error.lvclass">)
            n140 = call-dynamic "Create Logger.vi"("error in (no error)"=w392, "Logger.Error in"=w390) -> ("error out"=w391:errorcluster, "Logger.Error out"=w389:refnum<class "Logger.Error.lvclass">)  [unwired: 8 in]
            n141 = Bundle By Name(cluster=w387, "SelfRef"=w389) -> (w388:T3)
            n142 = call <vilib>:"Add State(s) to Queue__jki_lib_state_machine.vi"("State(s) in (\"\")"=w395) -> ("States Out"=w394:string)  [unwired: 14 in]
          }
          frame "Logger: Stop Error Logger" {
            n143 = Unbundle By Name(w396) -> ("SelfRef"=w399:refnum<class "Logger.Error.lvclass">)
            n144 = call-dynamic "Destroy Logger.vi"("error in (no error)"=w398, "Logger.Error in"=w399) -> ("error out"=w397:errorcluster)  [unwired: 8 in, 1 out]
            n145 = call <vilib>:"Add State(s) to Queue__jki_lib_state_machine.vi"("State(s) in (\"\")"=w402) -> ("States Out"=w401:string)  [unwired: 14 in]
          }
          frame "Logger: Log Error" {
            n146 = Unbundle By Name(w416) -> ("SelfRef"=w412:refnum<class "Logger.Error.lvclass">, "error to log"=w414:errorcluster)
            n147 = call-dynamic "Read path.vi"("error in (no error)"=w409, "Logger in"=w412) -> ("error out"=w410:errorcluster, "path"=w411:path)  [unwired: 7 in, 1 out]
            n148 = call "Error Cluster to Array.vi"("error in (no error)"=w414) -> ("Error Array"=w413:string[])  [unwired: 10 in]
            n149 = call-poly <vilib>:"Write Delimited Spreadsheet.vi"("file path (dialog if empty)"=w411, "1D data"=w413, "append to file? (new file:F)"=TRUE, "error in (no error)"=w410) -> ("error out"=w405:errorcluster)  [unwired: 10 in, 1 out]
            n150 = Get Date/Time In Seconds() -> (seconds since 1Jan1904=w407:timestamp)
            n151 = Format Into String(error in=w405, "Error Logged", w407) -> (resulting string=w406:string, error out=w404:errorcluster)  [unwired: 2 in]
            n152 = call <userlib>:"State History.vi"("Current State"=w406) -> ("History"=→"Status":string)  [unwired: 10 in]
            n153 = call <vilib>:"Add State(s) to Queue__jki_lib_state_machine.vi"("State(s) in (\"\")"=w419) -> ("States Out"=w418:string)  [unwired: 14 in]
          }
        }
      }
    }
    frame Error {
    }
  }
  n154 = call-parent "Process.vi"("error in"=w5, "Logger"=w4) -> ("error out"=w2:errorcluster, "Logger out"=→"Logger.Error out":refnum<class "Logger.Error.lvclass">)  [unwired: 8 in]
  n155 = Merge Errors(w2, w1) -> (→"error out":errorcluster)
